vi "TS Acq Stop.vi"(8 "error in (no error)":errorcluster, 11 "HTS Test Stand in":refnum<class "HTS Test Stand.lvclass">) -> (0 "error out":errorcluster, 3 "HTS Test Stand out":refnum<class "HTS Test Stand.lvclass">)   [LabVIEW 2019, in "Test Stands.lvlib" / "HTS Test Stand.lvclass"]
uses:
  HTS Test Stand.lvclass
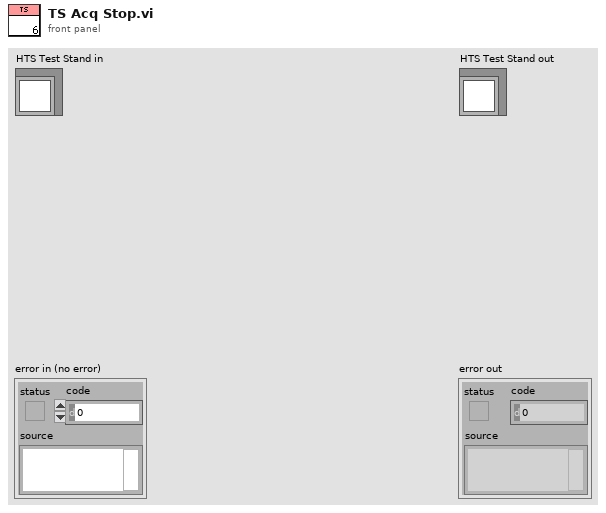
[diagram p1: front panel]
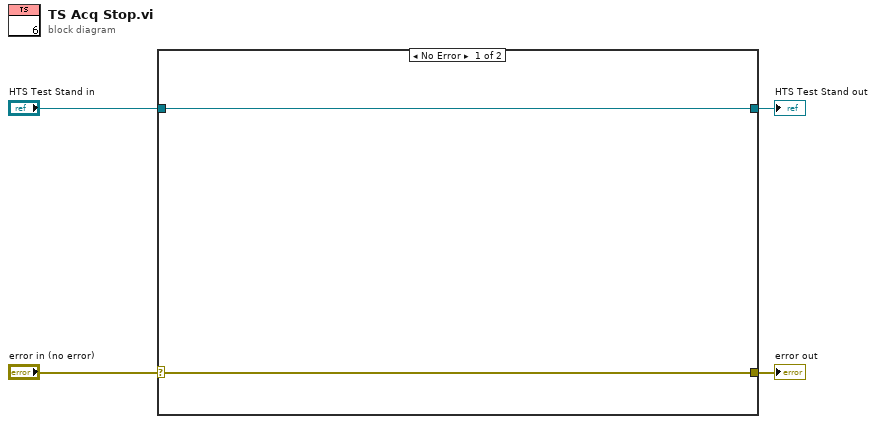
[diagram p0: block diagram]
diagram:
  n1 = case shown="No Error" "error in (no error)" {
    selector: "error in (no error)" -> [w5 w8]
    tunnel: [w5 w8] -> w1
    tunnel: [w6 w7] -> w3
    tunnel: "HTS Test Stand in" -> [w6 w7]
    frame No Error {
    }
    frame Error {
    }
  }
  "error out" <- w1
  "HTS Test Stand out" <- w3
